vi "Serialize - Text.vi"(8 "error in":errorcluster, 11 "SOAP Data in":refnum<class "SOAP Data.lvclass">) -> (0 "error out":errorcluster, 2 "Serialized Text":string, 3 "SOAP Data out":refnum<class "SOAP Data.lvclass">)   [LabVIEW 2017, in "Controller.lvlib" / "SOAP Data.lvclass"]
uses:
  SOAP Data.lvclass
  SOAP Data.lvclass/SOAP Data.ctl
  <vilib>/MSR Consulting, LLC/General Reuse/Data/Data.lvclass
  Heater Data/Heater Data.lvclass
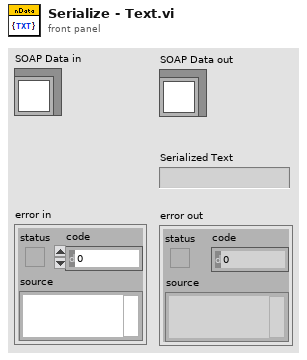
[diagram p1: front panel]
types:
  T1 = cluster{"pas_cell_1":sgl, "pas_cell_2":sgl, "pas_las_head_1":sgl, "pas_las_head_2":sgl, "box_exit":sgl, "crd_heater":sgl, "box_inlet":sgl, "crd_laser_head":sgl, "cjc":sgl, "autozero":sgl}
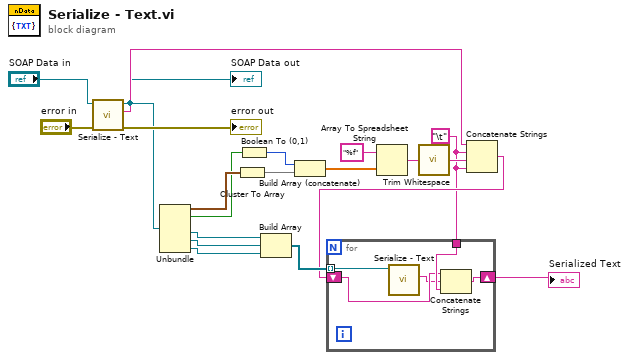
[diagram p0: block diagram]
diagram:
  w1 = "\t"
  n1 = call-parent "Serialize - Text.vi"("error in"="error in", "Data in"="SOAP Data in") -> ("error out"=→"error out":errorcluster, "Serialized Text"=w12:string, "Data out"=w10:refnum<class "SOAP Data.lvclass">)  [unwired: 7 in]
  "SOAP Data out" <- w10
  n2 = Unbundle(w10) -> (w9:T1, w8:bool, w7:refnum<class "Heater Data.lvclass">, w6:refnum<class "Heater Data.lvclass">, w5:refnum<class "Heater Data.lvclass">)  [unwired: 1 out]
  n3 = Cluster To Array(cluster=w9) -> (array=w18:sgl[])
  n4 = Boolean To (0,1)(Boolean=w8) -> (0, 1=w19:i16)
  n5 = Build Array(w7, w6, w5) -> (w4:refnum<class "Heater Data.lvclass">[])
  n6 = Build Array (concatenate)(w19, w18) -> (w17:sgl[])
  n7 = Array To Spreadsheet String(array=w17, 3:"%f" ("format string")) -> (spreadsheet string=w16:string)  [unwired: 1 in]
  n8 = call <vilib>:"Trim Whitespace.vi"("string"=w16) -> ("trimmed string"=w11:string)  [unwired: 1 in]
  n9 = Concatenate Strings(w12, w1, w11, w1) -> (w3:string)
  n10 = for {
    tunnel: w4 -> [w25] mode=indexing
    shift-right: [w24] -> w2
    shift-left: w3 -> [w22]
    tunnel: w1 -> [w23]
    n11 = call-dynamic "Serialize - Text.vi"("Heater Data in"=w25) -> ("Serialized Text"=w21:string)  [unwired: 8 in, 2 out]
    n12 = Concatenate Strings(w22, w21, w23) -> (w24:string)
  }
  "Serialized Text" <- w2
